vi "Rec setModifiedData.vi"(4 "error in (no error)":errorcluster, 6 "data":T1, 7 "recordset reference":T3) -> (0 "error out":errorcluster, 3 "recordset reference out":T3)   [LabVIEW 2012, in "NI_Database_API_64.lvlib"]
doc: "This VI overwrites the data associated with the <B>Recordset</B> object reference and unlocks it for write access. If <B>error in</B> is set, the object is unlocked but its data will not be modified.\n\nIn order to use this VI, you must first successfully lock the object's data using the <B>Rec Get Data To Modify</B> VI.\n\n[GOOP 1.0/1.0]"
uses:
  NI_Database_API_64.lvlib
  Rec DataMembers.ctl
  Connection.llb/Conn ObjectReference.ctl
  Rec ObjectReference.ctl
  <vilib>/Utility/_goopsup.llb/GOOP Object Repository Method.ctl
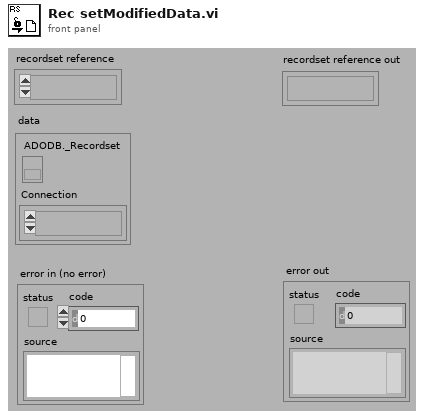
[diagram p1: front panel]
types:
  T1 = typedef "NI_Database_API_64.lvlib/Rec DataMembers.ctl" = cluster{"ADODB._Recordset":refnum<k7>, "Connection":T2}
  T2 = typedef "NI_Database_API_64.lvlib/Conn ObjectReference.ctl" = refnum<k1>
  T3 = typedef "NI_Database_API_64.lvlib/Rec ObjectReference.ctl" = refnum<k1>
  T4 = typedef "GOOP Object Repository Method.ctl" = enum16{"Create", "GetCopy", "GetModify", "Set", "Destroy", "Create Static", "Get All Refs", "Reset", "Get Statistics"}
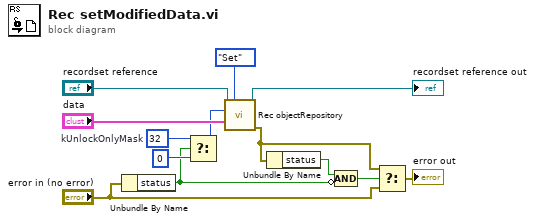
[diagram p0: block diagram]
diagram:
  w6 = 32  # kUnlockOnlyMask
  n1 = Unbundle By Name("error in (no error)") -> ("status"=w3:bool)
  n2 = Select(t=w6, s=w3, f=0 ("flags in")) -> (s? t:f=w4:i32)
  n3 = call "Rec objectRepository.vi"("recordset reference"="recordset reference", "method"=GOOP_Object_Repository_Method."Set", "flags in"=w4, "classDataIn"="data") -> ("recordset reference out"=→"recordset reference out":T3, "error out"=w10:errorcluster)  [unwired: 5 in, 5 out]
  n4 = Unbundle By Name(w10) -> ("status"=w2:bool)
  n5 = Compound Arithmetic op=AND(w2, invert w3) -> (w1:bool)
  n6 = Select(t=w10, s=w1, f="error in (no error)") -> (s? t:f=→"error out":errorcluster)
